vi "View STD Error.vi"(8 "error in":errorcluster caption="에러 입력(에러 없음)", 11 "Data":string[][](array[string])) -> (0 "error out":errorcluster caption="에러 출력")   [LabVIEW 2020]
uses:
  <vilib>/Utility/miscctls.llb/LVPoint32TypeDef.ctl
  Public/Polymorph/Sort_2D Str.vi
panel:
  in  "정렬":enum16{"오름차순", "내림차순"}(ring)
  out "원소":i32
  out "배열":i32[][](array[numeric])
  out "좌표":T1
  in  "List":i32[](listbox)
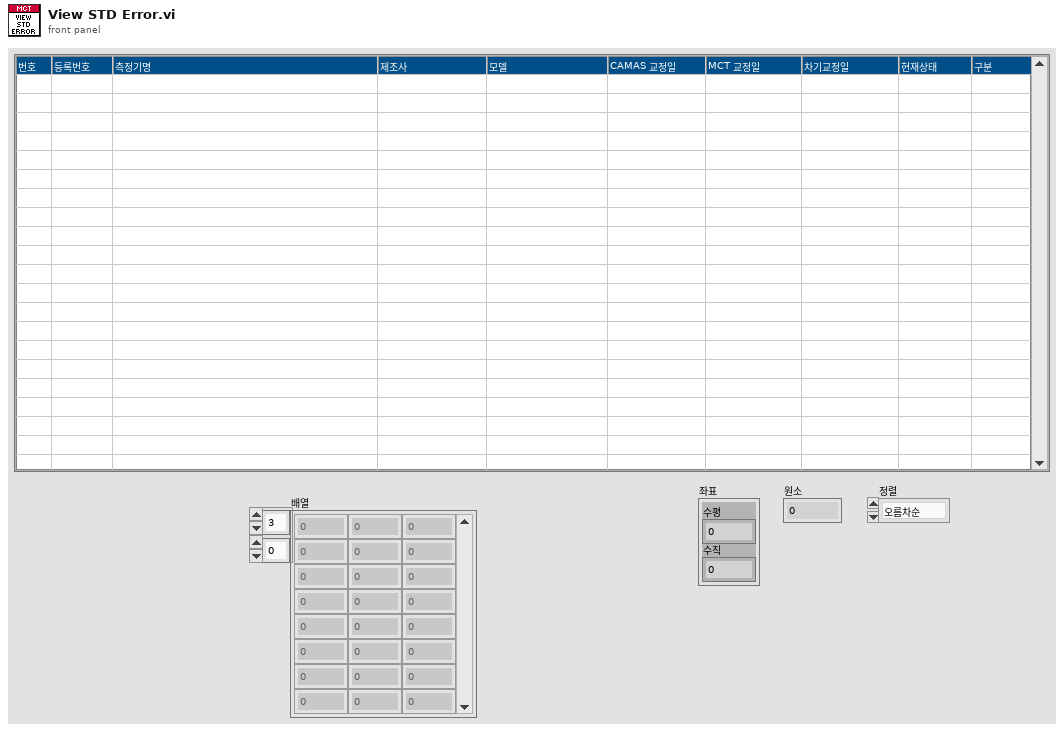
[diagram p1: front panel]
types:
  T1 = typedef "LVPoint32TypeDef.ctl" = cluster{"Horizontal":i32, "Vertical":i32}
  T2 = enum16{"Initialize", "Start", "Wait", "Sort", "Exit"}
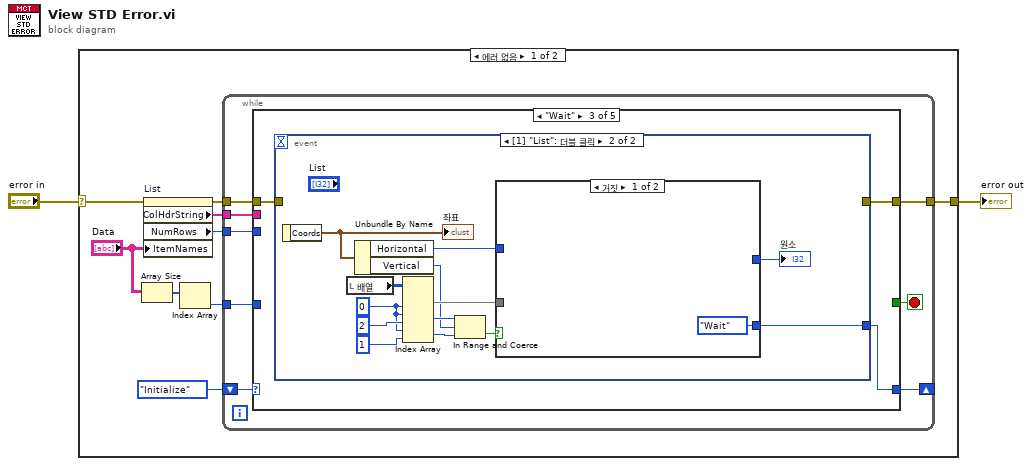
[diagram p0: block diagram]
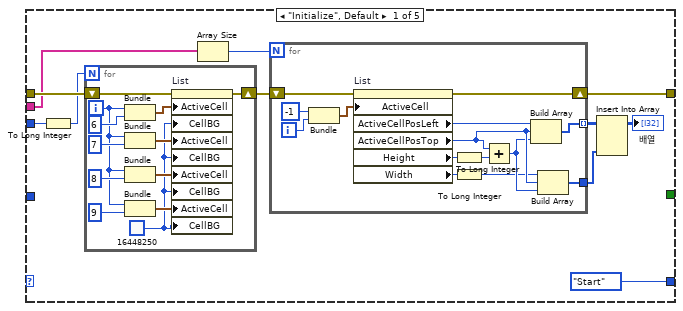
[diagram p2: hidden frame]
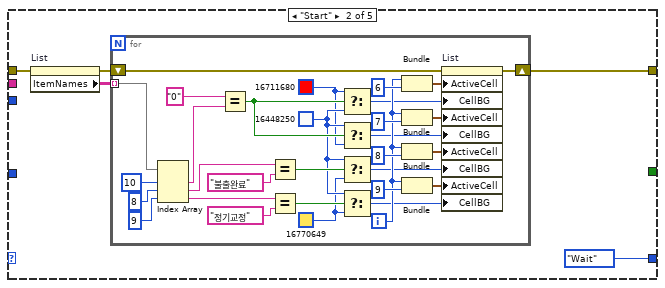
[diagram p3: hidden frame]
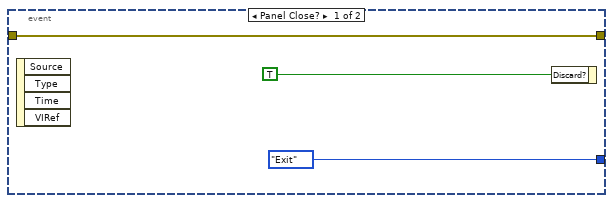
[diagram p4: hidden frame]
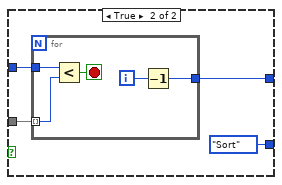
[diagram p5: hidden frame]
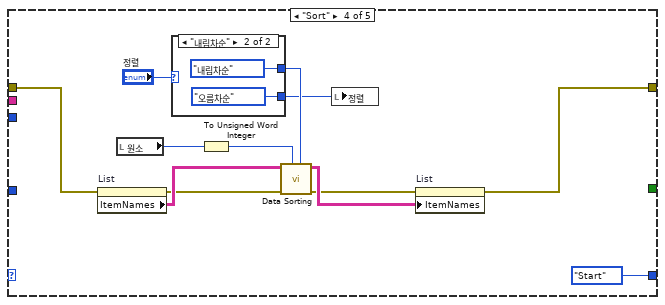
[diagram p6: hidden frame]
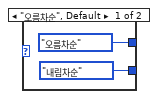
[diagram p7: hidden frame]
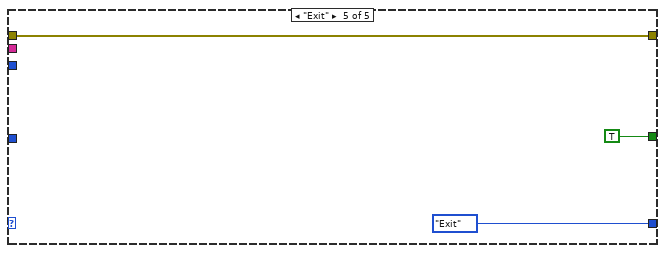
[diagram p8: hidden frame]
diagram:
  n1 = case shown="에러 없음" "error in" {
    selector: "error in" -> [w9 w141]
    tunnel: [w11 w141] -> w2
    frame No Error {
      n2 = Array Size(array="Data") -> (size(s)=w7:i32[])
      n3 = property on="List" class="MCListbox (엄격한)"(error in=w9, "ItemNames"="Data") -> (error out=w8:errorcluster, "ColHdrString"=w4:string[], "NumRows"=w5:u32)  [unwired: 1 in, 1 out]
      n4 = Index Array(array=w7) -> (element=w6:i32)  [unwired: 1 in]
      n5 = while {
        tunnel: w8 -> [w17]
        tunnel: [w18] -> w11
        shift-right: [w15] -> _
        shift-left: T2."Initialize" -> [w19]
        tunnel: w6 -> [w14]
        tunnel: w5 -> [w13]
        tunnel: w4 -> [w12]
        stop <- w16 stop-if-true
        n6 = case shown="\"Wait\"" w19 {
          tunnel: [w23 w60 w95 w126 w139] -> w18
          tunnel: w17 -> [w28 w59 w94 w133 w139]
          tunnel: [_ _ _ _ TRUE] -> w16
          tunnel: [T2."Start" T2."Wait" w93 T2."Start" T2."Exit"] -> w15
          tunnel: w14 -> [_ _ _ _ _]
          tunnel: w13 -> [w29 _ _ _ _]
          tunnel: w12 -> [w20 _ _ _ _]
          frame "Initialize", Default {
            n7 = To Long Integer(number=w29) -> (32bit integer=w27:i32)
            n8 = for {
              N: w27 -> [_]
              shift-right: [w55] -> w24
              shift-left: w28 -> [w56]
              i -> [w48]
              w45 = u32 16448250
              n9 = Bundle(w48, 6) -> (w54:cluster{i32, i32})  [unwired: 1 in]
              n10 = Bundle(w48, 7) -> (w52:cluster{i32, i32})  [unwired: 1 in]
              n11 = Bundle(w48, 8) -> (w47:cluster{i32, i32})  [unwired: 1 in]
              n12 = Bundle(w48, 9) -> (w46:cluster{i32, i32})  [unwired: 1 in]
              n13 = property on="List" class="MCListbox (엄격한)"(error in=w56, "ActiveCell"=w54, "CellBG"=w45, "ActiveCell"=w52, "CellBG"=w45, "ActiveCell"=w47, "CellBG"=w45, "ActiveCell"=w46, "CellBG"=w45) -> (error out=w55:errorcluster)  [unwired: 1 in, 1 out]
            }
            n14 = Array Size(array=w20) -> (size(s)=w21:i32)
            n15 = for {
              N: w21 -> [_]
              shift-right: [w43] -> w23
              shift-left: w24 -> [w44]
              tunnel: [w38] -> w26 mode=indexing
              tunnel: [w32] -> w25
              i -> [w42]
              n16 = Bundle(-1, w42) -> (w40:cluster{i32, i32})  [unwired: 1 in]
              n17 = property on="List" class="MCListbox (엄격한)"(error in=w44, "ActiveCell"=w40) -> (error out=w43:errorcluster, "ActiveCellPosLeft"=w39:i32, "ActiveCellPosTop"=w34:i32, "Height"=w37:u32, "Width"=w35:u32)  [unwired: 1 in, 1 out]
              n18 = To Long Integer(number=w37) -> (32bit integer=w36:i32)
              n19 = To Long Integer(number=w35) -> (32bit integer=w31:i32)
              n20 = Add(x=w34, y=w36) -> (x+y=w33:i32)
              n21 = Build Array(w39, w34, w33) -> (w38:i32[])
              n22 = Build Array(w31, w34, w33) -> (w32:i32[])
            }
            n23 = Insert Into Array(array=w26, new element=w25) -> (→"배열":i32[][])  [unwired: 2 in]
          }
          frame "Start" {
            n24 = property on="List" class="MCListbox (엄격한)"(error in=w59) -> (error out=w58:errorcluster, "ItemNames"=w57:string[][])  [unwired: 1 in, 1 out]
            n25 = for {
              shift-right: [w78] -> w60
              shift-left: w58 -> [w79]
              tunnel: w57 -> [w90] mode=indexing
              i -> [w77]
              w63 = u32 16711680
              w62 = u32 16770649
              w64 = u32 16448250
              n26 = Index Array(array=w90, index #1=10 ("인덱스"), index #2=8 ("인덱스"), index #3=9 ("인덱스")) -> (element #1=w68:string, element #2=w72:string, element #3=w71:string)
              n27 = Equal?(x="0", y=w68) -> (x = y?=w65:bool)
              n28 = Equal?(x=w72, y="불출완료") -> (x = y?=w74:bool)
              n29 = Equal?(x=w71, y="정기교정") -> (x = y?=w76:bool)
              n30 = Select(t=w63, s=w65, f=w64) -> (s? t:f=w67:u32)
              n31 = Select(t=w64, s=w65, f=w63) -> (s? t:f=w66:u32)
              n32 = Select(t=w64, s=w74, f=w62) -> (s? t:f=w73:u32)
              n33 = Select(t=w64, s=w76, f=w62) -> (s? t:f=w75:u32)
              n34 = Bundle(w77, 6) -> (w80:cluster{i32, i32})  [unwired: 1 in]
              n35 = Bundle(w77, 7) -> (w82:cluster{i32, i32})  [unwired: 1 in]
              n36 = Bundle(w77, 8) -> (w86:cluster{i32, i32})  [unwired: 1 in]
              n37 = Bundle(w77, 9) -> (w87:cluster{i32, i32})  [unwired: 1 in]
              n38 = property on="List" class="MCListbox (엄격한)"(error in=w79, "ActiveCell"=w80, "CellBG"=w67, "ActiveCell"=w82, "CellBG"=w66, "ActiveCell"=w86, "CellBG"=w73, "ActiveCell"=w87, "CellBG"=w75) -> (error out=w78:errorcluster)  [unwired: 1 in, 1 out]
            }
          }
          frame "Wait" {
            n39 = event shown="[1] \"List\": 더블 클릭" {
              selector: _ -> [_ _]
              dyn-events: _ -> [_ _]
              timeout: _ -> [_ _]
              tunnel: [w98 _] -> w95
              tunnel: w94 -> [w98 _]
              tunnel: [T2."Exit" w99] -> w93
              event Panel Close? {
                n40 = event-data() -> ()  [unwired: 1 in, 4 out]
                n41 = event-data("Discard?"=TRUE ("버림?")) -> ()  [unwired: 1 in, 1 out]
              }
              event "List": Double Click {
                w105 = 0 ("비활성화된 인덱스 (열)")
                n42 = event-data() -> ("Coords"=w109:T1)  [unwired: 1 in]
                "좌표" <- w109
                n43 = local read "배열"() -> (w111:i32[][])
                n44 = Unbundle By Name(w109) -> ("Horizontal"=w108:i32, "Vertical"=w101:i32)
                n45 = Index Array(array=w111, index (col) #1=w105, index (row) #2=w105, index (col) #2=2 ("비활성화된 인덱스 (열)"), index (row) #3=w105, index (col) #3=1 ("비활성화된 인덱스 (열)")) -> (element #1=w110:i32[], element #2=w103:i32, element #3=w102:i32)  [unwired: 1 in]
                n46 = In Range and Coerce(upper limit=w103, x=w101, lower limit=w102) -> (In Range?=w100:bool)  [unwired: 1 out]
                n47 = case shown="거짓" w100 {
                  tunnel: w110 -> [_ w116]
                  tunnel: w108 -> [_ w115]
                  tunnel: [_ w114] -> w107
                  tunnel: [T2."Wait" T2."Sort"] -> w99
                  frame False {
                  }
                  frame True {
                    n48 = for {
                      tunnel: w116 -> [w120] mode=indexing
                      tunnel: w115 -> [w119]
                      tunnel: [w117] -> w114
                      i -> [w121]
                      stop <- w118 stop-if-true
                      n49 = Less?(x=w119, y=w120) -> (x < y?=w118:bool)
                      n50 = Decrement(x=w121) -> (x-1=w117:i32)
                    }
                  }
                }
                "원소" <- w107
              }
            }
          }
          frame "Sort" {
            n51 = property on="List" class="MCListbox (엄격한)"(error in=w133) -> (error out=w129:errorcluster, "ItemNames"=w132:string[][])  [unwired: 1 in, 1 out]
            n52 = local read "원소"() -> (w131:i32)
            n53 = case shown="\"내림차순\"" "정렬" {
              tunnel: [enum16{"오름차순", "내림차순"}."오름차순" ("정렬") enum16{"오름차순", "내림차순"}."내림차순" ("정렬")] -> w124
              tunnel: [enum16{"오름차순", "내림차순"}."내림차순" ("정렬") enum16{"오름차순", "내림차순"}."오름차순" ("정렬")] -> w123
              frame "오름차순", Default {
              }
              frame "내림차순" {
              }
            }
            n54 = To Unsigned Word Integer(number=w131) -> (unsigned 16bit integer=w130:u16)
            n55 = call-poly "Data Sorting.vi"("정렬"=w124, "기준열"=w130, "error in (no error)"=w129, "Data in"=w132) -> ("error out"=w127:errorcluster, "Data out"=w128:string[][])  [unwired: 6 in]
            n56 = local write "정렬"(w123) -> ()
            n57 = property on="List" class="MCListbox (엄격한)"(error in=w127, "ItemNames"=w128) -> (error out=w126:errorcluster)  [unwired: 1 in, 1 out]
          }
          frame "Exit" {
          }
        }
      }
    }
    frame Error {
    }
  }
  "error out" <- w2
